vi "Get Joint Array.vi"(8 "error in":errorcluster, 10 "Tree Elements":T1(array[cluster]), 11 "Scene In":refnum<vi>) -> (0 "error out":errorcluster, 2 "Joint Array":T2(array[cluster]), 3 "Scene Out":refnum<vi>)   [LabVIEW 2020]
doc: "This VI created an array of all the joints"
uses:
  <vilib>/picture/3D Picture Control/NI_3D Picture Control.lvlib
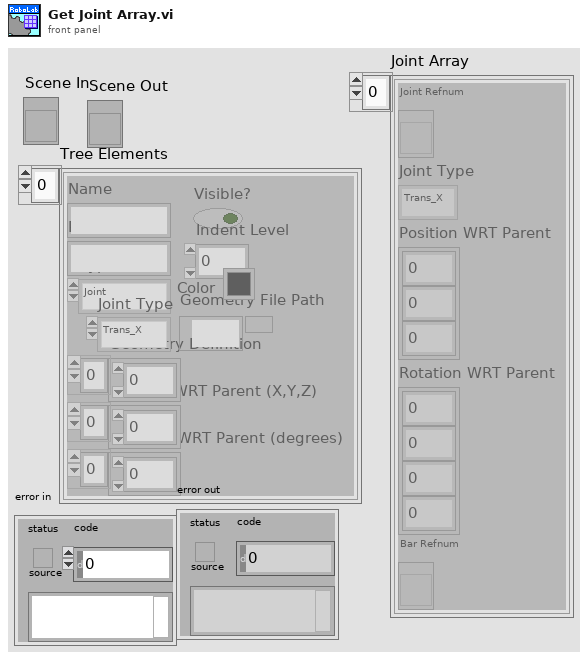
[diagram p1: front panel]
types:
  T1 = cluster{"Name":string, "Parent":string, "Type":enum16{"Joint", "Box", "Cylinder", "Cone", "Sphere", "ASE File", "VRML File", "STL File", "Space"}, "Visible?":bool, "Geometry Definition":dbl[], "Position WRT Parent (X,Y,Z)":dbl[], "Rotation WRT Parent (degrees)":dbl[], "Joint Type":enum16{"Trans_X", "Trans_Y", "Trans_Z", "Rot_X", "Rot_Y", "Rot_Z", "None"}, "Geometry File Path":path, "Indent Level":i32, "Color":u32}[]
  T2 = cluster{"Joint Refnum":refnum<vi>, "Joint Type":enum16{"Trans_X", "Trans_Y", "Trans_Z", "Rot_X", "Rot_Y", "Rot_Z", "None"}, "Position WRT Parent":dbl[], "Rotation WRT Parent":dbl[], "Bar Refnum":refnum<vi>}[]
  T3 = cluster{"Joint Refnum":refnum<vi>, "Joint Type":enum16{"Trans_X", "Trans_Y", "Trans_Z", "Rot_X", "Rot_Y", "Rot_Z", "None"}, "Position WRT Parent":dbl[], "Rotation WRT Parent":dbl[], "Bar Refnum":refnum<vi>}
  T4 = enum16{"Joint", "Box", "Cylinder", "Cone", "Sphere", "ASE File", "VRML File", "STL File", "Space"}
  T5 = enum16{"Trans_X", "Trans_Y", "Trans_Z", "Rot_X", "Rot_Y", "Rot_Z", "None"}
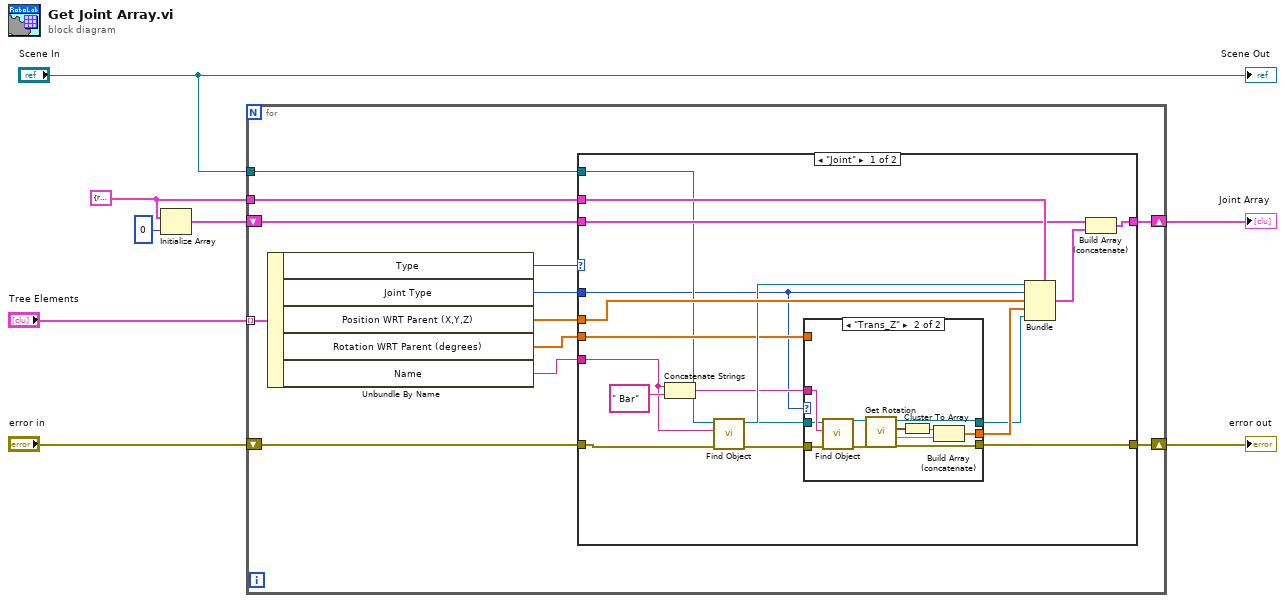
[diagram p0: block diagram]
diagram:
  w7 = T3 {"Joint Refnum"=refnum, "Joint Type"=enum."Trans_X", "Position WRT Parent"=[], "Rotation WRT Parent"=[], "Bar Refnum"=refnum} ("Joints")
  n1 = Initialize Array(w7, 0 ("dimension size")) -> (w6:T2)
  n2 = for {
    tunnel: "Scene In" -> [w20]
    tunnel: "Tree Elements" -> [w19] mode=indexing
    shift-right: [w15] -> w8
    shift-left: w6 -> [w16]
    tunnel: w7 -> [w17]
    shift-right: [w14] -> w2
    shift-left: "error in" -> [w18]
    n3 = Unbundle By Name(w19) -> ("Type"=w12:T4, "Joint Type"=w11:T5, "Position WRT Parent (X,Y,Z)"=w10:dbl[], "Rotation WRT Parent (degrees)"=w9:dbl[], "Name"=w13:string)
    n4 = case shown="\"Joint\"" w12 {
      tunnel: w20 -> [w25 _]
      tunnel: w13 -> [w31 _]
      tunnel: w18 -> [w27 w53]
      tunnel: [w23 w53] -> w14
      tunnel: w11 -> [w21 _]
      tunnel: w17 -> [w37 _]
      tunnel: w16 -> [w35 w52]
      tunnel: [w34 w52] -> w15
      tunnel: w10 -> [w33 _]
      tunnel: w9 -> [w29 _]
      frame "Joint" {
        n5 = Concatenate Strings(w31, " Bar" ("string")) -> (w26:string)
        n6 = call <vilib>:"Find Object.vi"("error in (no error)"=w27, "Object Name"=w31, "Scene Refnum"=w25) -> ("error out"=w24:errorcluster, "Object Refnum"=w30:refnum<vi>)  [unwired: 7 out]
        n7 = case shown="\"Trans_Z\"" w21 {
          tunnel: w29 -> [w40 _]
          tunnel: [w40 w48] -> w28
          tunnel: w26 -> [_ w47]
          tunnel: w25 -> [w38 w46]
          tunnel: w24 -> [w39 w44]
          tunnel: [w39 w42] -> w23
          tunnel: [w38 w41] -> w22
          frame Default {
          }
          frame "Trans_Z" {
            n8 = call <vilib>:"Find Object.vi"("error in (no error)"=w44, "Object Name"=w47, "Scene Refnum"=w46) -> ("error out"=w43:errorcluster, "Object Refnum"=w45:refnum<vi>)  [unwired: 7 out]
            n9 = call <vilib>:"Get Rotation.vi"("error in (no error)"=w43, "Scene Object"=w45) -> ("error out"=w42:errorcluster, "Angle"=w49:sgl, "Axis"=w51:cluster{"X":sgl, "Y":sgl, "Z":sgl}, "Scene Object"=w41:refnum<vi>)  [unwired: 6 in]
            n10 = Cluster To Array(cluster=w51) -> (array=w50:sgl[])
            n11 = Build Array (concatenate)(w50, w49) -> (w48:sgl[])
          }
        }
        n12 = Bundle(cluster=w37, "Joint Refnum"=w30, "Joint Type"=w21, "Position WRT Parent"=w33, "Rotation WRT Parent"=w28, "Bar Refnum"=w22) -> (w36:T3)
        n13 = Build Array (concatenate)(w35, w36) -> (w34:T2)
      }
      frame Default {
      }
    }
  }
  "Joint Array" <- w8
  "error out" <- w2
  "Scene Out" <- "Scene In"
